vi "ReadSetupFile.vi"(8 "Error In":errorcluster, 11 "Setup File":path) -> (0 "Error Out":errorcluster, 3 "Setup":T1={"Chamber Name"="", "Log Folder Path"=path "", "Heater"={"COM Port"=0, "Setpoint"=0.0, "Standby?"=FALSE}, "MFC"={"COM Port"=0, "Timeout (msec)"=0, "Setpoint"=0.0, "Valve State"=enum."Automatic", "Gas"=enum."Air", "Units"=enum."scc/m", "Serial Number"="", "Firmware Version"=""}})   [LabVIEW 2012]
uses:
  Setup.ctl
  HeaterConfiguration.ctl
  MFCConfiguration.ctl
  libs/Sierra-M100/Public/Controls/ValveState.ctl
  libs/Sierra-M100/Public/Controls/Gas.ctl
  libs/Sierra-M100/Public/Controls/Units.ctl
  <vilib>/Utility/config.llb/Read Key (String).vi
  <vilib>/Utility/config.llb/Read Key (Path).vi
  <vilib>/Utility/config.llb/Read Key (I32).vi
  <vilib>/Utility/config.llb/NI_LVConfig.lvlib
  libs/Sierra-M100/Sierra-M100.lvlib
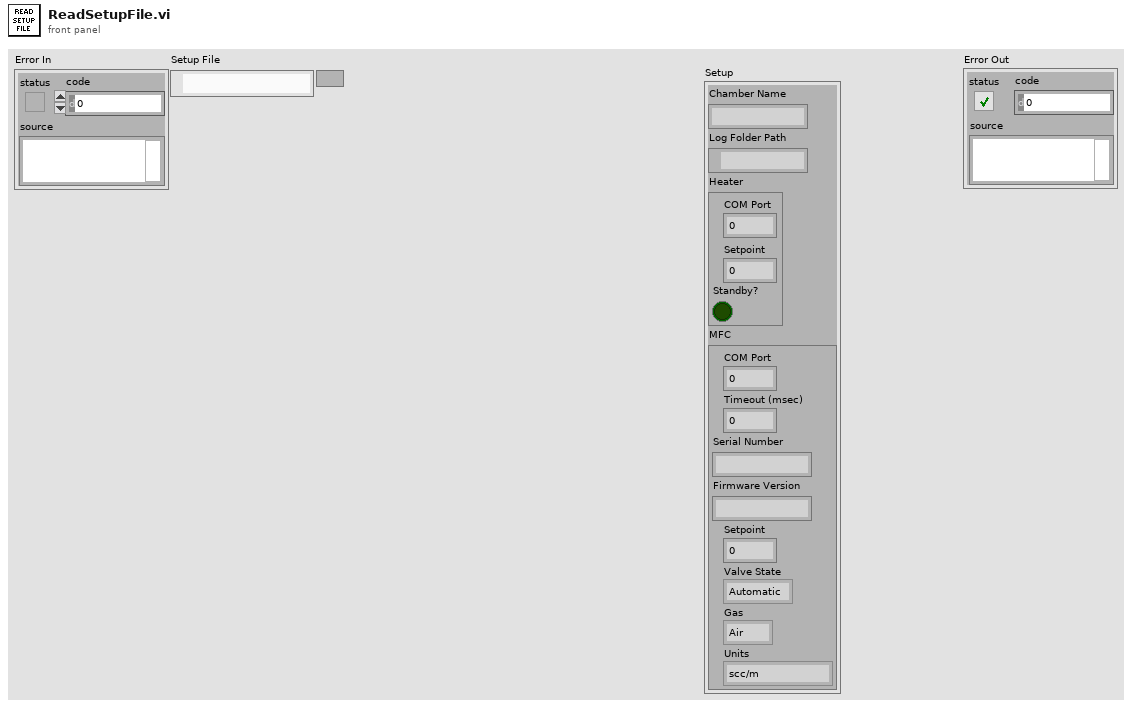
[diagram p1: front panel]
types:
  T1 = typedef "Setup.ctl" = cluster{"Chamber Name":string, "Log Folder Path":path, "Heater":T2, "MFC":T3}
  T2 = typedef "HeaterConfiguration.ctl" = cluster{"COM Port":u8, "Setpoint":dbl, "Standby?":bool}
  T3 = typedef "MFCConfiguration.ctl" = cluster{"COM Port":u32, "Timeout (msec)":u32, "Setpoint":dbl, "Valve State":T4, "Gas":T5, "Units":T6, "Serial Number":string, "Firmware Version":string}
  T4 = typedef "Sierra-M100.lvlib/ValveState.ctl" = enum16{"Automatic", "Closed", "Purge"}
  T5 = typedef "Sierra-M100.lvlib/Gas.ctl" = enum16{"Air", "Argon", "CO2", "CO", "Helium", "Hydrogen", "Methane", "Nitrogen", "Nitrous Oxide", "Oxygen"}
  T6 = typedef "Sierra-M100.lvlib/Units.ctl" = enum16{"scc/s", "scc/m", "scc/H", "Ncc/s", "Ncc/m", "Ncc/H", "SCF/s", "SCF/m", "SCF/H", "NM3/s", "NM3/m", "NM3/H", "SM3/s", "SM3/m", "SM3/H", "sl/s", "sl/m", "sl/H", "NL/s", "NL/m", "Nl/H", "g/s", "g/m", "g/H", "kg/s", "kg/m", "kg/H", "lb/s", "lb/m", "lb/H"}
  T7 = typedef "NI_LVConfig.lvlib/Config Data RefNum.ctl" = refnum<k1>
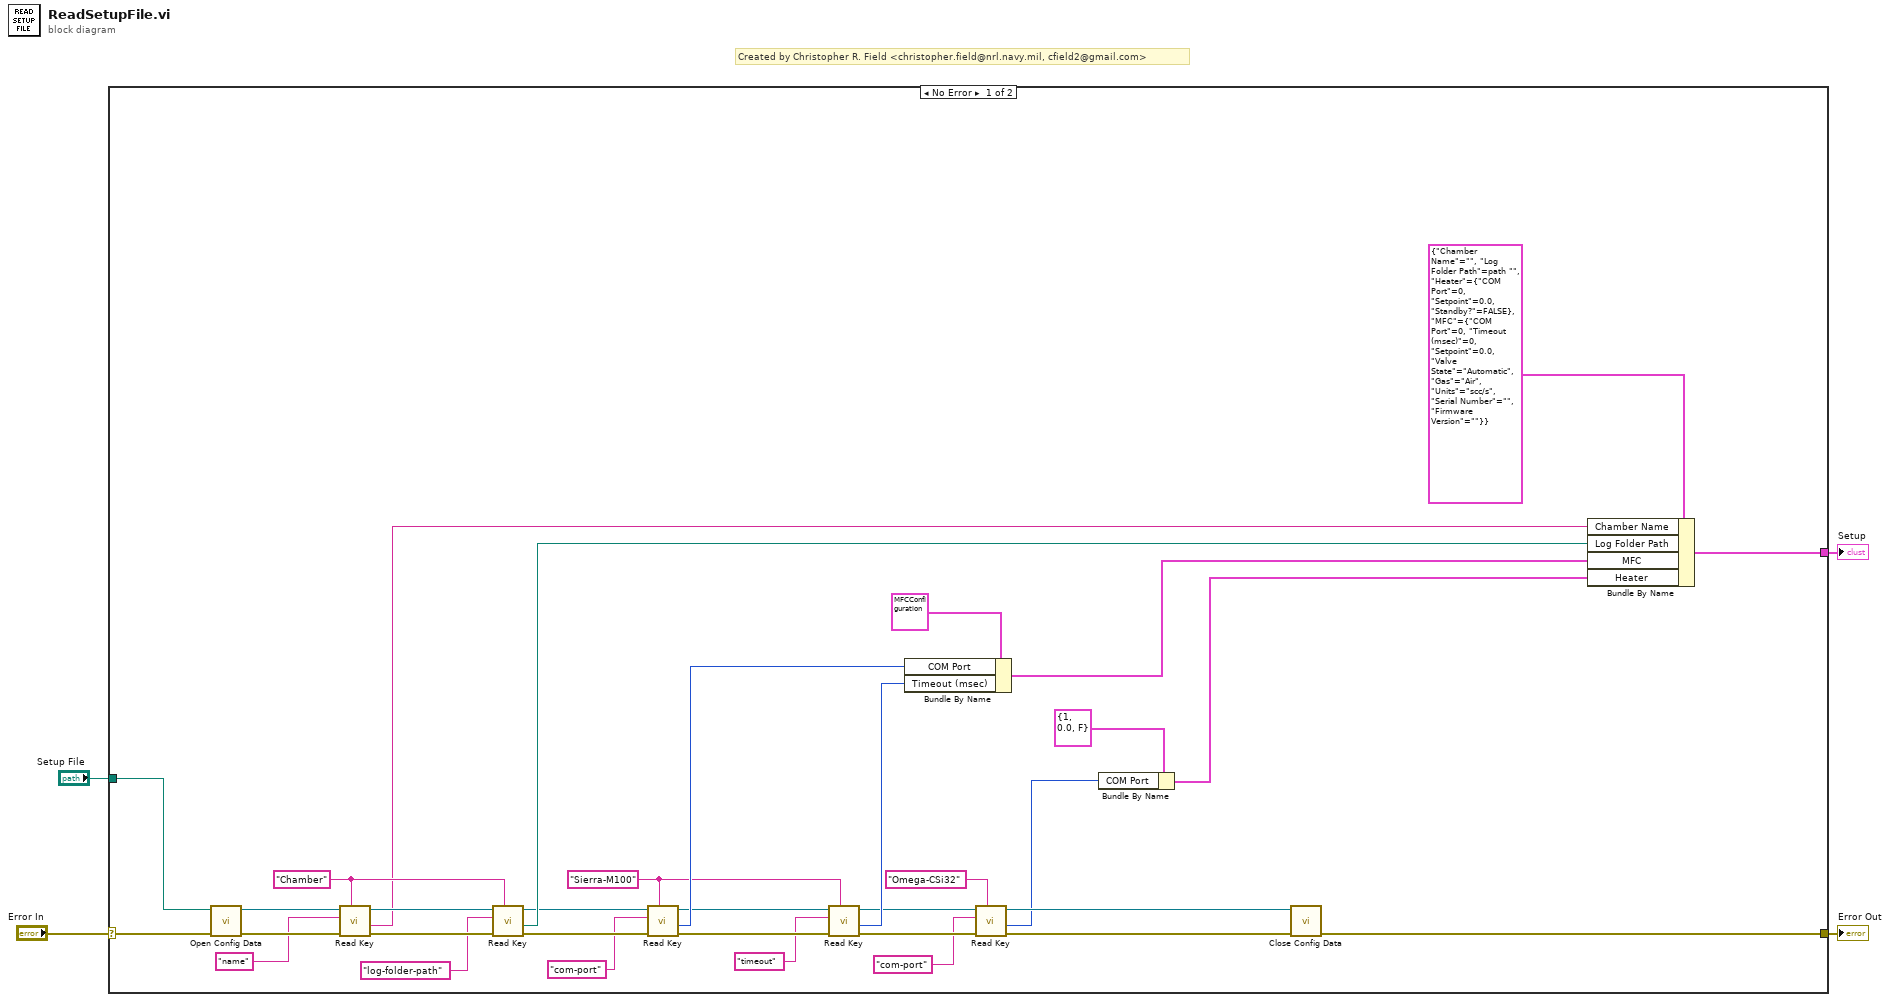
[diagram p0: block diagram]
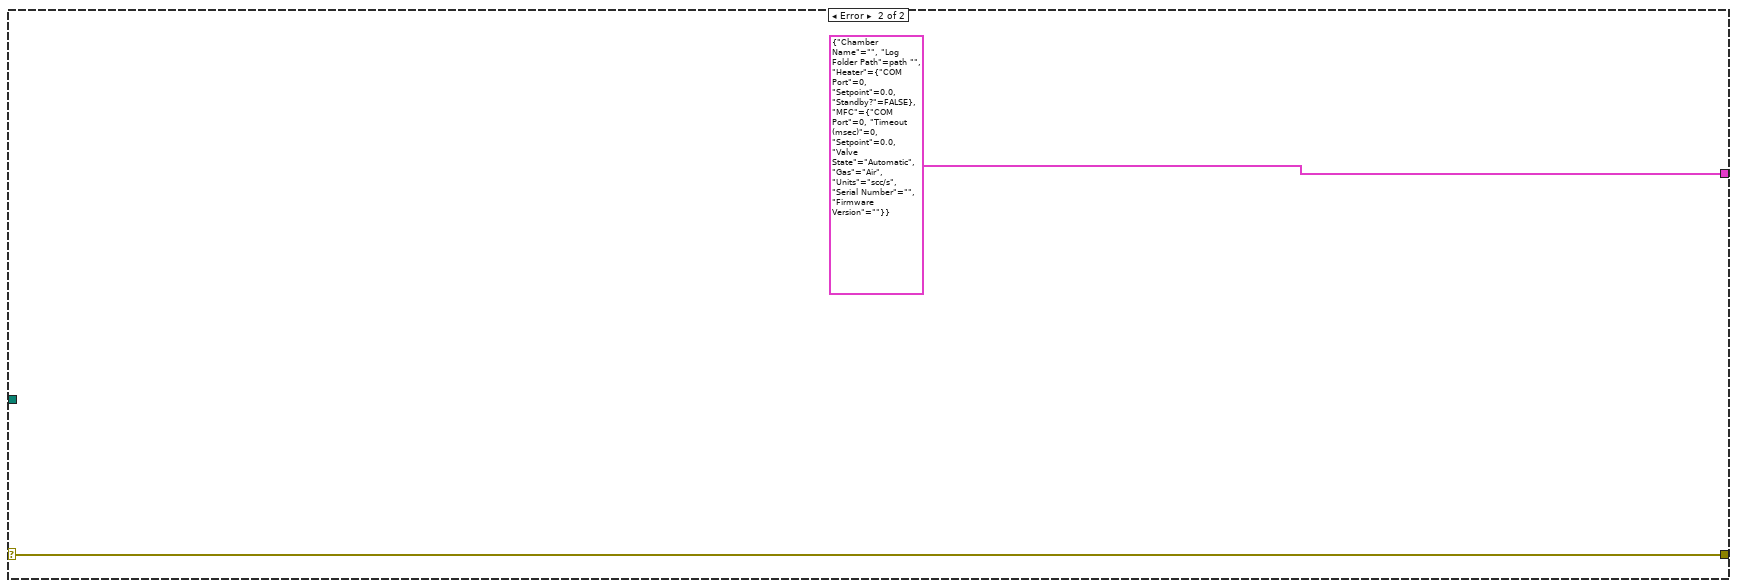
[diagram p2: hidden frame]
diagram:
  # "Created by Christopher R. Field <christopher.field@nrl.navy.mil, cfield2@gmail.com>"
  n1 = case shown="No Error" "Error In" {
    selector: "Error In" -> [w38 w40]
    tunnel: "Setup File" -> [w32 _]
    tunnel: [w34 T1 {"Chamber Name"="", "Log Folder Path"=path "", "Heater"={"COM Port"=0, "Setpoint"=0.0, "Standby?"=FALSE}, "MFC"={"COM Port"=0, "Timeout (msec)"=0, "Setpoint"=0.0, "Valve State"=enum."Automatic", "Gas"=enum."Air", "Units"=enum."scc/s", "Serial Number"="", "Firmware Version"=""}} ("Sample Chamber Configuration")] -> w1
    tunnel: [w25 w40] -> w2
    frame No Error {
      w17 = "Sierra-M100" ("section")
      w29 = "Chamber" ("section")
      n2 = call <vilib>:"Open Config Data.vi"("error in (no error)"=w38, "configuration file path"=w32) -> ("error out"=w36:errorcluster, "refnum"=w37:T7)  [unwired: 7 in, 1 out]
      n3 = call-poly <vilib>:"Read Key.vi"("section"=w29, "error in (no error)"=w36, "key"="name", "refnum"=w37) -> ("error out"=w30:errorcluster, "value"=w27:string, "refnum out"=w31:T7)  [unwired: 4 in, 1 out]
      n4 = call-poly <vilib>:"Read Key.vi"("section"=w29, "error in (no error)"=w30, "key"="log-folder-path", "refnum"=w31) -> ("error out"=w21:errorcluster, "value"=w26:path, "refnum out"=w22:T7)  [unwired: 4 in, 1 out]
      n5 = call-poly <vilib>:"Read Key.vi"("section"=w17, "error in (no error)"=w21, "key"="com-port", "refnum"=w22) -> ("error out"=w16:errorcluster, "value"=w20:i32, "refnum out"=w18:T7)  [unwired: 4 in, 1 out]
      n6 = call-poly <vilib>:"Read Key.vi"("section"=w17, "error in (no error)"=w16, "key"="timeout", "refnum"=w18) -> ("error out"=w11:errorcluster, "value"=w14:i32, "refnum out"=w12:T7)  [unwired: 4 in, 1 out]
      n7 = Bundle By Name(cluster=T3 {"COM Port"=1, "Timeout (msec)"=100, "Setpoint"=0.0, "Valve State"=enum."Automatic", "Gas"=enum."Air", "Units"=enum."scc/m", "Serial Number"="", "Firmware Version"=""} ("MFC Configuration"), "COM Port"=w20, "Timeout (msec)"=w14) -> (w23:T3)
      n8 = call-poly <vilib>:"Read Key.vi"("section"="Omega-CSi32", "error in (no error)"=w11, "key"="com-port", "refnum"=w12) -> ("error out"=w8:errorcluster, "value"=w6:i32, "refnum out"=w9:T7)  [unwired: 4 in, 1 out]
      n9 = Bundle By Name(cluster=T2 {"COM Port"=1, "Setpoint"=0.0, "Standby?"=FALSE} ("Heater Configuration"), "COM Port"=w6) -> (w5:T2)
      n10 = call <vilib>:"Close Config Data.vi"("error in (no error)"=w8, "refnum"=w9) -> ("error out"=w25:errorcluster)  [unwired: 8 in, 1 out]
      n11 = Bundle By Name(cluster=T1 {"Chamber Name"="", "Log Folder Path"=path "", "Heater"={"COM Port"=0, "Setpoint"=0.0, "Standby?"=FALSE}, "MFC"={"COM Port"=0, "Timeout (msec)"=0, "Setpoint"=0.0, "Valve State"=enum."Automatic", "Gas"=enum."Air", "Units"=enum."scc/s", "Serial Number"="", "Firmware Version"=""}} ("Sample Chamber Configuration"), "Chamber Name"=w27, "Log Folder Path"=w26, "MFC"=w23, "Heater"=w5) -> (w34:T1)
    }
    frame Error {
    }
  }
  "Error Out" <- w2
  "Setup" <- w1
